vi "5-1.vi"() -> ()   [LabVIEW 2019, in "5.lvlib"]
uses:
  5.lvlib
panel:
  out "sum":i16
  out "Array":i32[][](array[numeric])
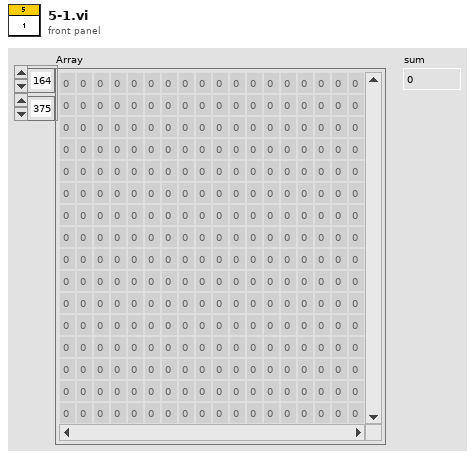
[diagram p1: front panel]
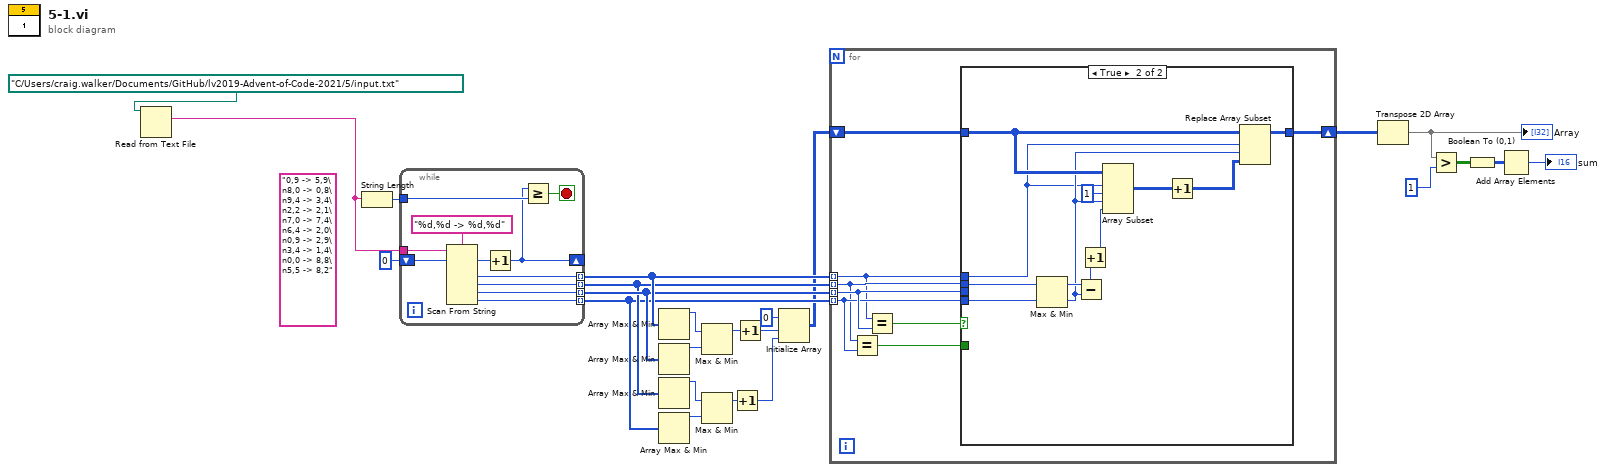
[diagram p0: block diagram]
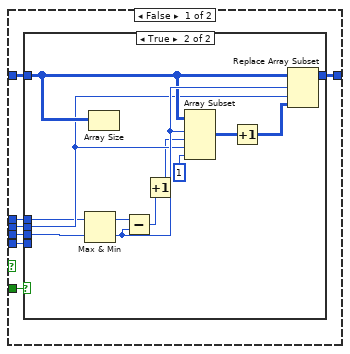
[diagram p2: hidden frame]
diagram:
  (unwired) "0,9 -> 5,9\n8,0 -> 0,8\n9,4 -> 3,4\n2,2 -> 2,1\n7,0 -> 7,4\n6,4 -> 2,0\n0,9 -> 2,9\n3,4 -> 1,4\n0,0 -> 8,8\n5,5 -> 8,2"
  n1 = Read from Text File(file (use dialog)=path "C:/Users/craig.walker/Documents/GitHub/lv2019-Advent-of-Code-2021/5/input.txt" ("file path (dialog if empty)")) -> (text=w1:string)  [unwired: 3 in, 3 out]
  n2 = String Length(string=w1) -> (length=w23:i32)
  n3 = while {
    tunnel: w1 -> [w35]
    shift-right: [w25] -> _
    shift-left: u32 0 -> [w34]
    tunnel: w23 -> [w27]
    tunnel: [w31] -> w20 mode=indexing
    tunnel: [w30] -> w12 mode=indexing
    tunnel: [w29] -> w19 mode=indexing
    tunnel: [w28] -> w11 mode=indexing
    stop <- w33 stop-if-true
    n4 = Scan From String(format string="%d,%d -> %d,%d", input string=w35, initial scan location=w34) -> (offset past scan=w26:u32, output 1=w31:i32, output 2=w30:i32, output 3=w29:i32, output 4=w28:i32)  [unwired: 5 in, 2 out]
    n5 = Increment(x=w26) -> (x+1=w25:u32)
    n6 = Greater Or Equal?(x=w25, y=w27) -> (x >= y?=w33:bool)
  }
  n7 = Array Max & Min(array=w20) -> (max value=w18:i32)  [unwired: 3 out]
  n8 = Array Max & Min(array=w19) -> (max value=w17:i32)  [unwired: 3 out]
  n9 = Array Max & Min(array=w12) -> (max value=w13:i32)  [unwired: 3 out]
  n10 = Array Max & Min(array=w11) -> (max value=w14:i32)  [unwired: 3 out]
  n11 = Max & Min(x=w18, y=w17) -> (max(x,y)=w15:i32)  [unwired: 1 out]
  n12 = Max & Min(x=w13, y=w14) -> (max(x,y)=w10:i32)  [unwired: 1 out]
  n13 = Increment(x=w10) -> (x+1=w7:i32)
  n14 = Increment(x=w15) -> (x+1=w8:i32)
  n15 = Initialize Array(0, w8, w7) -> (w9:i32[][])
  n16 = for {
    shift-right: [w42] -> w21
    shift-left: w9 -> [w43]
    tunnel: w20 -> [w36] mode=indexing
    tunnel: w12 -> [w37] mode=indexing
    tunnel: w19 -> [w41] mode=indexing
    tunnel: w11 -> [w38] mode=indexing
    n17 = Equal?(x=w37, y=w38) -> (x = y?=w39:bool)
    n18 = Equal?(x=w36, y=w41) -> (x = y?=w40:bool)
    n19 = case shown="True" w40 {
      tunnel: w37 -> [w50 w66]
      tunnel: w41 -> [w49 _]
      tunnel: w43 -> [w48 w75]
      tunnel: [w47 w69] -> w42
      tunnel: w39 -> [w46 _]
      tunnel: w36 -> [w45 w67]
      tunnel: w38 -> [w44 w68]
      frame False {
        n20 = case shown="True" w46 {
          tunnel: w50 -> [_ w56]
          tunnel: w49 -> [_ w54]
          tunnel: w48 -> [w51 w57]
          tunnel: [w51 w61] -> w47
          tunnel: w45 -> [_ w55]
          tunnel: w44 -> [_ _]
          frame False {
          }
          frame True {
            n21 = Max & Min(x=w55, y=w54) -> (max(x,y)=w63:i32, min(x,y)=w58:i32)
            n22 = Array Size(array=w57) -> ()  [unwired: 1 out]
            n23 = Subtract(x=w63, y=w58) -> (x-y=w59:i32)
            n24 = Increment(x=w59) -> (x+1=w52:i32)
            n25 = Array Subset(array=w57, index (row)=w58, length (row)=w52, index (col)=w56, length (col)=1 ("length")) -> (w62:i32[][])
            n26 = Increment(x=w62) -> (x+1=w53:i32[][])
            n27 = Replace Array Subset(array=w57, new element=w53, index (row)=w58, index (col)=w56) -> (w61:i32[][])
          }
        }
      }
      frame True {
        n28 = Max & Min(x=w66, y=w68) -> (max(x,y)=w74:i32, min(x,y)=w70:i32)
        n29 = Subtract(x=w74, y=w70) -> (x-y=w72:i32)
        n30 = Increment(x=w72) -> (x+1=w64:i32)
        n31 = Array Subset(array=w75, index (row)=w67, length (row)=1 ("length"), index (col)=w70, length (col)=w64) -> (w71:i32[][])
        n32 = Increment(x=w71) -> (x+1=w65:i32[][])
        n33 = Replace Array Subset(array=w75, new element=w65, index (row)=w67, index (col)=w70) -> (w69:i32[][])
      }
    }
  }
  n34 = Transpose 2D Array(2D array=w21) -> (transposed array=w6:i32[][])
  "Array" <- w6
  n35 = Greater?(x=w6, y=1) -> (0:w4:bool[][])
  n36 = Boolean To (0,1)(Boolean=w4) -> (0, 1=w3:i16[][])
  n37 = Add Array Elements(numeric array=w3) -> (sum=→"sum":i16)
